vi "IMAQdx_getAttribute_I64.vi"(3 "error in (no error)":errorcluster, 4 "Attribute Name":string, 5 "IMAQdx Session":T1) -> (0 "error out":errorcluster, 1 "IMAQdx Attribute":variant, 2 "dup IMAQdx Session":T1)   [LabVIEW 2014, in "HGF_VisionTools.lvlib"]
doc: "This VI reads IMAQdx attribute value of type I64 and its properties. Value is returned as Variant and properties as Variant attributes."
uses:
  HGF_VisionTools.lvlib
  <resource>/objmgr/imaqdx.rc
  <vilib>/userdefined/High Color/IMAQdx.ctl
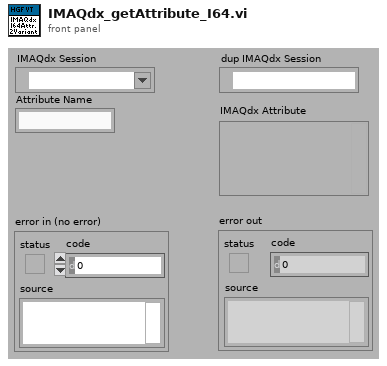
[diagram p1: front panel]
types:
  T1 = typedef "IMAQdx.ctl" = refnum<k21>
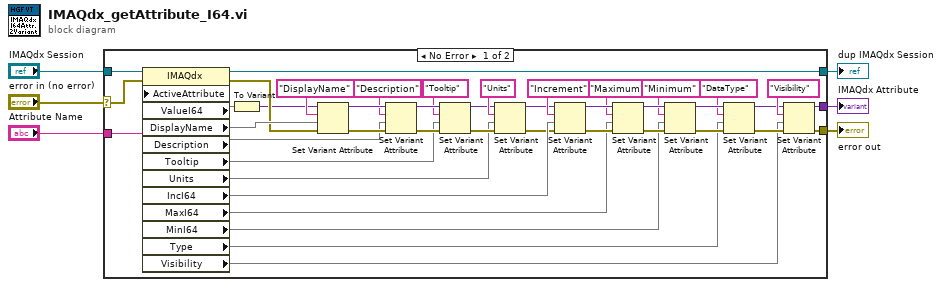
[diagram p0: block diagram]
diagram:
  n1 = case shown="No Error" "error in (no error)" {
    selector: "error in (no error)" -> [w7 w51]
    tunnel: "IMAQdx Session" -> [w49 w50]
    tunnel: "Attribute Name" -> [w48 _]
    tunnel: [w47 w50] -> w4
    tunnel: [w15 _] -> w3
    tunnel: [w14 w51] -> w2
    frame No Error {
      n2 = property class="IMAQdx"(reference=w49, error in=w7, "ActiveAttribute"=w48) -> (reference out=w47:T1, error out=w44:errorcluster, "ValueI64"=w43, "DisplayName"=w45, "Description"=w25, "Tooltip"=w24, "Units"=w8, "IncI64"=w23, "MaxI64"=w22, "MinI64"=w21, "Type"=w20, "Visibility"=w16)
      n3 = To Variant(anything=w43) -> (Variant=w42:variant)
      n4 = Set Variant Attribute(Variant=w42, name="DisplayName", value=w45, error in=w44) -> (Variant out=w41:variant, error out=w32:errorcluster)  [unwired: 1 out]
      n5 = Set Variant Attribute(Variant=w41, name="Description", value=w25, error in=w32) -> (Variant out=w40:variant, error out=w33:errorcluster)  [unwired: 1 out]
      n6 = Set Variant Attribute(Variant=w40, name="Tooltip", value=w24, error in=w33) -> (Variant out=w9:variant, error out=w10:errorcluster)  [unwired: 1 out]
      n7 = Set Variant Attribute(Variant=w9, name="Units", value=w8, error in=w10) -> (Variant out=w12:variant, error out=w11:errorcluster)  [unwired: 1 out]
      n8 = Set Variant Attribute(Variant=w12, name="Increment", value=w23, error in=w11) -> (Variant out=w39:variant, error out=w34:errorcluster)  [unwired: 1 out]
      n9 = Set Variant Attribute(Variant=w39, name="Maximum", value=w22, error in=w34) -> (Variant out=w38:variant, error out=w35:errorcluster)  [unwired: 1 out]
      n10 = Set Variant Attribute(Variant=w38, name="Minimum", value=w21, error in=w35) -> (Variant out=w37:variant, error out=w36:errorcluster)  [unwired: 1 out]
      n11 = Set Variant Attribute(Variant=w37, name="DataType", value=w20, error in=w36) -> (Variant out=w17:variant, error out=w18:errorcluster)  [unwired: 1 out]
      n12 = Set Variant Attribute(Variant=w17, name="Visibility", value=w16, error in=w18) -> (Variant out=w15:variant, error out=w14:errorcluster)  [unwired: 1 out]
    }
    frame Error {
    }
  }
  "IMAQdx Attribute" <- w3
  "dup IMAQdx Session" <- w4
  "error out" <- w2
